vi "poly_set_xwav_attribute.vi"(1 "attributes (none)":variant, 3 "xwave in":T1={"attributes"=variant, "X"={"start"=0.0, "delta"=0.0, "units"="index", "dim"="au"}, "Y"={"data"=[], "units"="au"}}) -> (0 "xwave out":T1={"attributes"=variant, "X"={"start"=0.0, "delta"=0.0, "units"="index", "dim"="au"}, "Y"={"data"=[], "units"="au"}})   [LabVIEW 2015, in "_xwav_polys.lvlib"]
uses:
  _xwav_polys.lvlib
  xwav.ctl
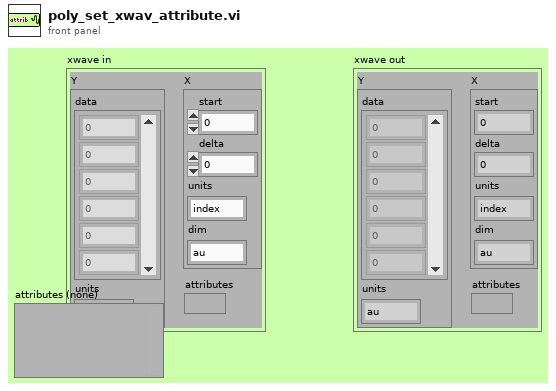
[diagram p1: front panel]
types:
  T1 = typedef "xwav.ctl" = cluster{"attributes":variant, "X":cluster{"start":dbl, "delta":dbl, "units":string, "dim":string}, "Y":cluster{"data":dbl[], "units":string}}
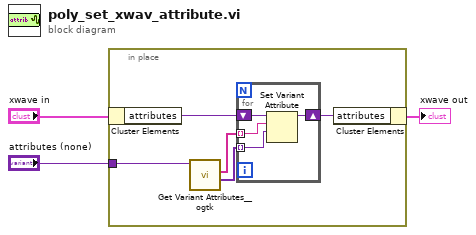
[diagram p0: block diagram]
diagram:
  n1 = in-place {
    in-place-border: "attributes (none)" -> [w6]
    n2 = in-place-cluster #1("xwave in") -> ("attributes"=w8:variant)
    n3 = call <userlib>:"Get Variant Attributes__ogtk.vi"("Variant"=w6) -> ("value(s)"=w5:variant[], "names"=w4:string[])  [unwired: 3 in, 2 out]
    n4 = for {
      tunnel: w5 -> [w10] mode=indexing
      tunnel: w4 -> [w11] mode=indexing
      shift-right: [w12] -> w7
      shift-left: w8 -> [w9]
      n5 = Set Variant Attribute(Variant=w9, name=w11, value=w10) -> (Variant out=w12:variant)  [unwired: 1 in, 2 out]
    }
    n6 = in-place-cluster #1("attributes"=w7) -> (→"xwave out":T1)
  }
